vi "Launch Nested Views.vi"(8 "error in (no error)":errorcluster, 9 "View Labels (optional)":string[](array[string]), 10 "Viewables":refnum<class "IViewable.lvclass">[](array[class]), 11 "Popup ViewManager in":refnum<class "Popup ViewManager.lvclass">) -> (0 "error out":errorcluster, 3 "Popup ViewManager out":refnum<class "Popup ViewManager.lvclass">)   [LabVIEW 2017, in "Popup ViewManager.lvlib" / "Popup ViewManager.lvclass"]
uses:
  <vilib>/gpm_packages/@cs/popup-viewmanager/Source/Popup ViewManager/Popup ViewManager.lvclass
  C:/Program Files/National Instruments/LabVIEW 2017/vi.lib/ActorFramework/Actor/Actor.lvclass
  C:/Program Files/National Instruments/LabVIEW 2017/vi.lib/gpm_packages/@cs/mva-viewable/Source/IViewable/IViewable/IViewable.lvclass
  <vilib>/gpm_packages/@cs/mva-viewable/Source/IViewable/IViewable/IViewable.lvclass
  C:/Program Files/National Instruments/LabVIEW 2017/vi.lib/gpm_packages/@cs/mva-core/Source/IObserver/IObserver/IObserver.lvclass
  <vilib>/gpm_packages/@cs/mva-viewable/Source/IViewable/IViewable/IViewable.lvclass/IViewable.ctl
  <vilib>/gpm_packages/@cs/mva-core/Source/IObserver/IObserver/IObserver.lvclass/IObserver.ctl
  <vilib>/gpm_packages/@cs/popup-viewmanager/Source/Popup ViewManager/Popup ViewManager.lvclass/Popup ViewManager.ctl
  <vilib>/gpm_packages/@cs/mva-viewable/Source/IViewable/IViewable/Write Application Style Reference.vi
  <vilib>/gpm_packages/@cs/mva-viewable/Source/IViewable/IViewable/Read Application Style Reference.vi
  <vilib>/gpm_packages/@cs/mva-core/Source/IObserver/IObserver/Transfer Observer Resources.vi
  <vilib>/ActorFramework/Actor/Actor.lvclass
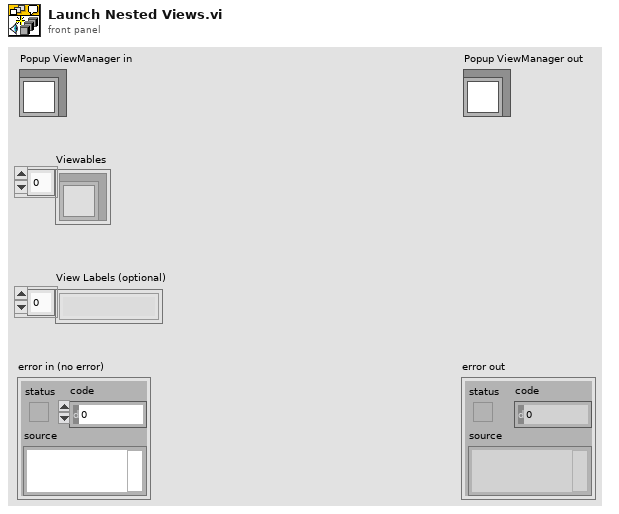
[diagram p1: front panel]
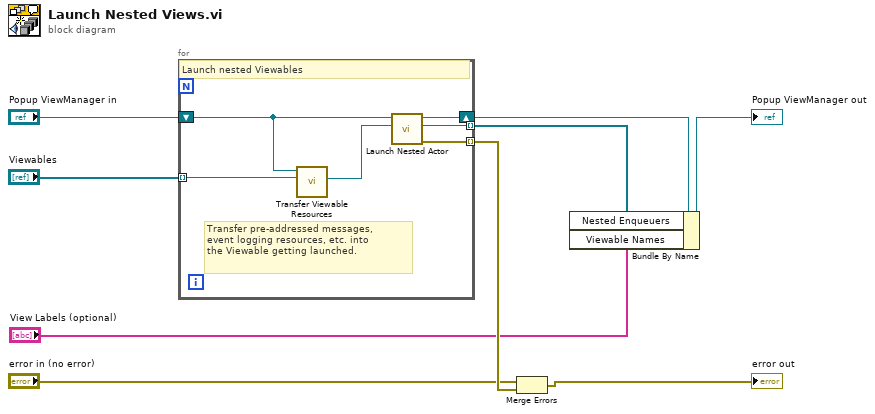
[diagram p0: block diagram]
diagram:
  n1 = for {
    shift-right: [w15] -> w3
    shift-left: "Popup ViewManager in" -> [w11]
    tunnel: "Viewables" -> [w14] mode=indexing
    tunnel: [w13] -> w6 mode=indexing
    tunnel: [w12] -> w9 mode=indexing
    # "Transfer pre-addressed messages,\nevent logging resources, etc. into\nthe Viewable getting launched."
    # "Launch nested Viewables"
    n2 = call <vilib>:"Transfer Viewable Resources.vi"("Recipient Viewable In"=w14, "Running Viewable"=w11) -> ("Recipient Viewable Out"=w10:refnum<class "IViewable.lvclass">)  [unwired: 9 in]
    n3 = call <vilib>:"Launch Nested Actor.vi"("Nested Actor"=w10, "Caller Actor in"=w11) -> ("error out"=w12:errorcluster, "Nested Actor's Enqueuer"=w13:refnum<class "Message Enqueuer.lvclass">, "Caller Actor out"=w15:refnum<class "Popup ViewManager.lvclass">)  [unwired: 7 in]
  }
  n4 = Merge Errors("error in (no error)", w9) -> (→"error out":errorcluster)
  n5 = Bundle By Name(cluster=w3, "Nested Enqueuers"=w6, "Viewable Names"="View Labels (optional)") -> (→"Popup ViewManager out":refnum<class "Popup ViewManager.lvclass">)
